vi "Set TC Type.vi"(8 "error in (no error)":errorcluster, 10 "Thermocouple Type (4: K)":u32(ring)=4 items=["B", "C", "E", "J", "K", "L:Jdin", "N", "R", "S", "T", "U:Tdin", "X", "Y", "Z"], 11 "VISA resource name":refnum<visa-resource-name>) -> (0 "error out":errorcluster, 3 "VISA resource name out":refnum<visa-resource-name>)   [LabVIEW 2011, in "Fluke 5XXX Series Multicalibrators.lvlib"]
doc: "This VI sets the Thermocouple (TC) temperature sensor type. The TC type is used when the output is set to a temperature value with the FL5XCAL Get Output Values.vi and the temperature sensor type is set to TC with the FL5XCAL Set Temp Sensor Type.vi . When the thermocouple type is changed while simulating a temperature output, the temperature is changed to 0 °C. Once set, the Calibrator retains the TC type until power off or reset.\n\nNote:\n\nThis VI is available only for instrument models 5500A and 5520A."
uses:
  Fluke 5XXX Series Multicalibrators.lvlib
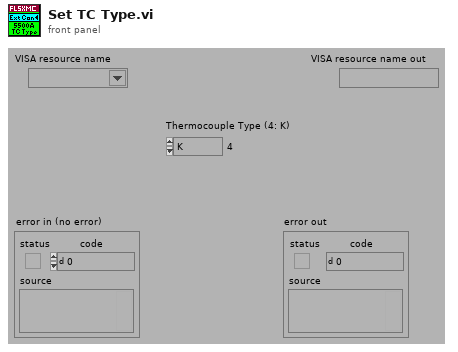
[diagram p1: front panel]
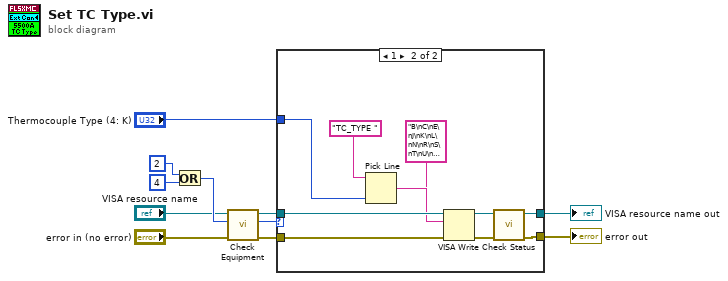
[diagram p0: block diagram]
diagram:
  n1 = Or(x=2 ("Numeric"), y=4 ("Numeric")) -> (x .or. y?=w8:i32)
  n2 = call "Check Equipment.vi"("error in (no error)"="error in (no error)", "Bit Mask"=w8, "VISA resource name"="VISA resource name") -> ("error out"=w11:errorcluster, "Present?"=w10:u32, "VISA resource name out"=w9:refnum<visa-resource-name>)  [unwired: 6 in]
  n3 = case shown="1" w10 {
    tunnel: "Thermocouple Type (4: K)" -> [_ w19]
    tunnel: [w12 w15] -> w1
    tunnel: w11 -> [w13 w22]
    tunnel: w9 -> [w12 w21]
    tunnel: [w13 w18] -> w2
    frame 0, Default {
    }
    frame 1 {
      n4 = Pick Line(string ("")="TC_TYPE " ("Reset Command"), multi-line string="B\nC\nE\nJ\nK\nL\nN\nR\nS\nT\nU\nX\nY\nZ", line index=w19) -> (output string=w20:string)
      n5 = VISA Write(VISA resource name=w21, write buffer=w20, error in (no error)=w22) -> (VISA resource name out=w16:refnum<visa-resource-name>, error out=w17:errorcluster)  [unwired: 1 out]
      n6 = call "Check Status.vi"("VISA resource name"=w16, "error in (no error)"=w17) -> ("VISA resource name out"=w15:refnum<visa-resource-name>, "error out"=w18:errorcluster)  [unwired: 12 in]
    }
  }
  "VISA resource name out" <- w1
  "error out" <- w2
